vi "task4.vi"() -> ()   [LabVIEW 2021]
uses:
  <vilib>/Utility/file.llb/Write Delimited Spreadsheet (DBL).vi
panel:
  in  "timeout (s)":dbl=10.0 format="%0.2f"
  out "Elapsed time (s)":dbl
  out "Sampling period (ms)":dbl
  out "Total number of samples":dbl
  in  "Sampling rate(Hz)":dbl
  in  "Total duration(s)":dbl
  out "Waveform Graph":dbl[](graph)
  in  "file path (dialog if empty)":path
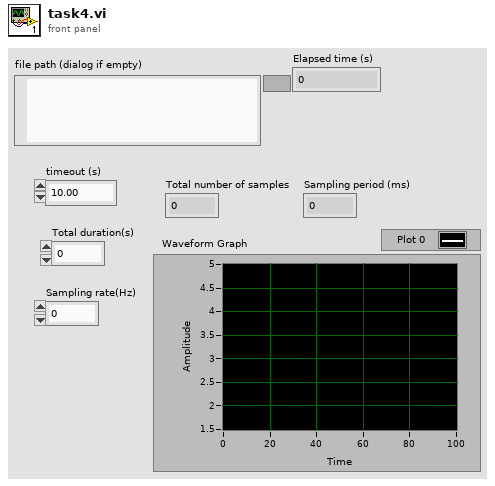
[diagram p1: front panel]
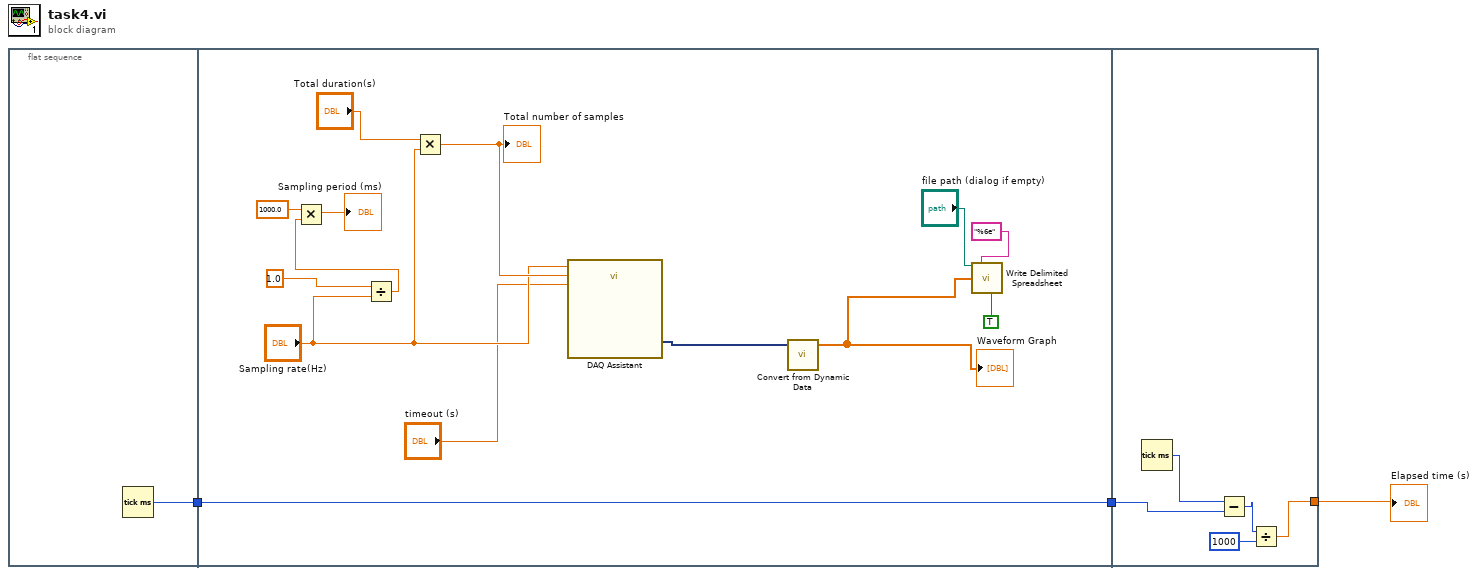
[diagram p0: block diagram]
diagram:
  n1 = flat-sequence {
    tunnel: [w4] -> w3
    tunnel: w3 -> [w10]
    tunnel: [w10] -> w2
    tunnel: w2 -> [w22]
    tunnel: [w19] -> w1
    frame #0 {
      n2 = Tick Count (ms)() -> (millisecond timer value=w4:u32)
    }
    frame #1 {
      n3 = Divide(x=1.0, y="Sampling rate(Hz)") -> (x/y=w12:dbl)
      n4 = Multiply(x=1000.0, y=w12) -> (x*y=→"Sampling period (ms)":dbl)
      n5 = Multiply(x="Total duration(s)", y="Sampling rate(Hz)") -> (x*y=w8:dbl)
      "Total number of samples" <- w8
      n6 = call "DAQ Assistant"("rate"="Sampling rate(Hz)", "number of samples"=w8, "timeout (s)"="timeout (s)") -> ("data"=w9:dynamicdata)  [unwired: 14 in, 2 out]
      n7 = call "Convert from Dynamic Data"("Dynamic Data Type"=w9) -> ("Array"=w6:dbl[])  [unwired: 3 in]
      "Waveform Graph" <- w6
      n8 = call-poly <vilib>:"Write Delimited Spreadsheet.vi"("file path (dialog if empty)"="file path (dialog if empty)", "format (%.3f)"="%6e", "1D data"=w6, "transpose? (no:F)"=TRUE) -> ()  [unwired: 10 in, 2 out]
    }
    frame #2 {
      n9 = Tick Count (ms)() -> (millisecond timer value=w23:u32)
      n10 = Subtract(x=w23, y=w22) -> (x-y=w21:u32)
      n11 = Divide(x=w21, y=u32 1000) -> (x/y=w19:dbl)
    }
  }
  "Elapsed time (s)" <- w1
